vi "Create.vi"(8 "error in (no error)":errorcluster) -> (0 "error out":errorcluster, 3 "queue out":refnum<queue>)   [LabVIEW 2016, in "System Queue.lvlib"]
uses:
  System Queue.lvlib
  Control_Queue Data.ctl
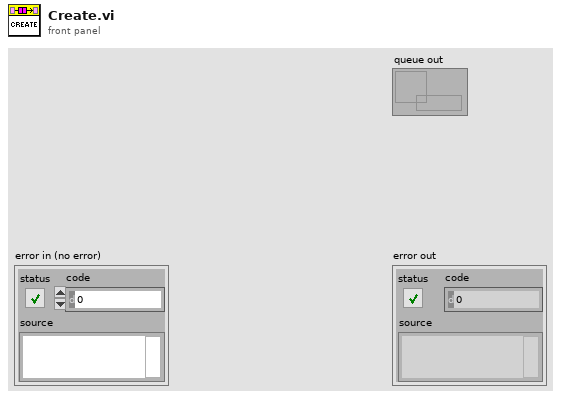
[diagram p1: front panel]
types:
  T1 = typedef "System Queue.lvlib/Control_Queue Data.ctl" = cluster{"Command":string, "Data":variant}
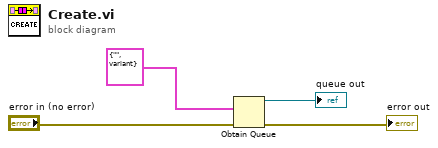
[diagram p0: block diagram]
diagram:
  n1 = Obtain Queue(element data type=T1 {"Command"="", "Data"=variant} ("Queue Data"), error in (no error)="error in (no error)") -> (queue out=→"queue out":refnum<queue>, error out=→"error out":errorcluster)  [unwired: 3 in, 1 out]
